vi "Init Interface.vi"(8 "error in":errorcluster, 9 "Config Section":string, 10 "hse-config":refnum<class "config-base.lvclass">, 11 "DB-Interface in":refnum<class "DB-Interface.lvclass">) -> (0 "error out":errorcluster, 3 "DB-Interface out":refnum<class "DB-Interface.lvclass">)   [LabVIEW 2022 SP3, in "hse-db.lvlib" / "DB-Interface.lvclass"]
doc: "____\nHAMPEL SOFTWARE ENGINEERING v1.4.0 (2023-12-19 09:52)"
uses:
  DB-Interface.lvclass
  hse-libraries/Source/hse-configuration/config-base/config-base.lvclass
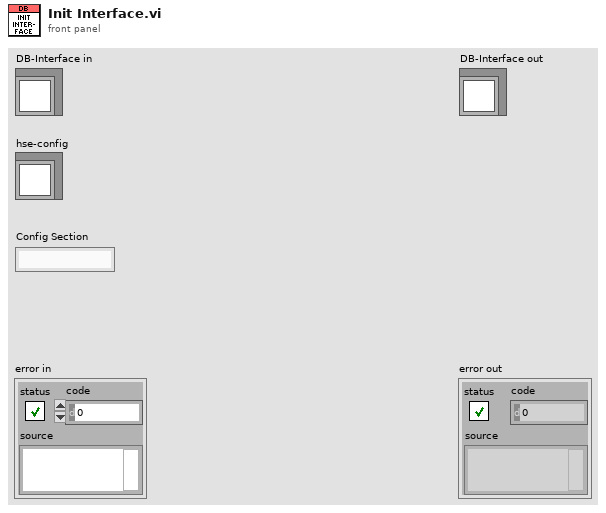
[diagram p1: front panel]
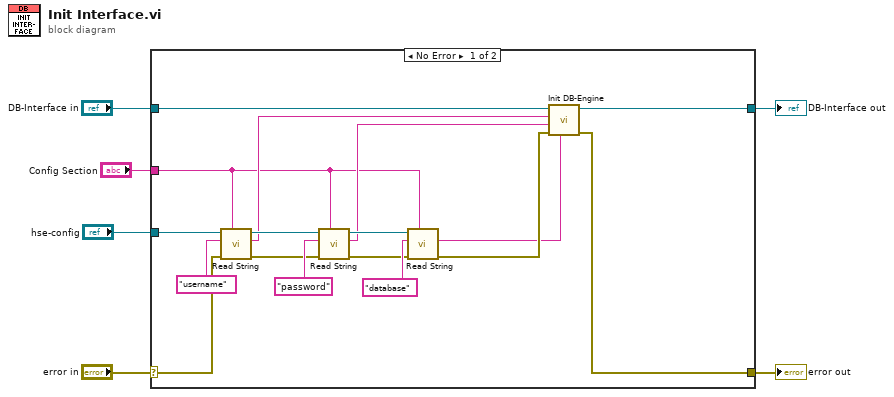
[diagram p0: block diagram]
diagram:
  n1 = case shown="No Error" "error in" {
    selector: "error in" -> [w23 w25]
    tunnel: [w21 w25] -> w5
    tunnel: [w19 w24] -> w3
    tunnel: "DB-Interface in" -> [w20 w24]
    tunnel: "hse-config" -> [w11 _]
    tunnel: "Config Section" -> [w7 _]
    frame No Error {
      n2 = call-dynamic "Read String.vi"("Section"=w7, "error in"=w23, "Key"="username", "config-base in"=w11) -> ("error out"=w12:errorcluster, "Value"=w10:string, "config-base out"=w13:refnum<class "config-base.lvclass">)  [unwired: 5 in]
      n3 = call-dynamic "Read String.vi"("Section"=w7, "error in"=w12, "Key"="password", "config-base in"=w13) -> ("error out"=w16:errorcluster, "Value"=w9:string, "config-base out"=w17:refnum<class "config-base.lvclass">)  [unwired: 5 in]
      n4 = call-dynamic "Read String.vi"("Section"=w7, "error in"=w16, "Key"="database", "config-base in"=w17) -> ("error out"=w22:errorcluster, "Value"=w8:string)  [unwired: 5 in, 1 out]
      n5 = call-dynamic "Init DB-Engine.vi"("Database"=w8, "error in"=w22, "Password"=w9, "User"=w10, "DB-Engine in"=w20) -> ("error out"=w21:errorcluster, "DB-Engine out"=w19:refnum<class "DB-Interface.lvclass">)  [unwired: 5 in]
    }
    frame Error {
    }
  }
  "error out" <- w5
  "DB-Interface out" <- w3
